vi "Msg To.vi"() -> (3 "Event Teardown Msg out":refnum<class "Event Teardown Msg.lvclass">)   [LabVIEW 2021, in "Event Teardown.lvlib" / "Event Teardown Msg.lvclass"]
uses:
  Event Teardown Msg.lvclass
  Event Teardown Msg.lvclass/Event Teardown Msg.ctl
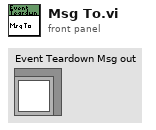
[diagram p1: front panel]
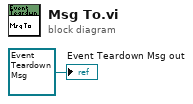
[diagram p0: block diagram]
diagram:
  "Event Teardown Msg out" <- refnum<class "Event Teardown Msg.lvclass"> refnum ("Event Teardown Msg out")
